vi "CalculateHaversineDirection.vi"(10 "Target Waypoint":cluster{"Longitude":dbl, "Latitude":dbl} {"Latitude" format="%#_8g"}, 11 "Robot Position":cluster{"Longitude":dbl, "Latitude":dbl}) -> (2 "polar angle":dbl)   [LabVIEW 2011]
panel:
  out "Robot Latitude":dbl
  out "Robot Longitude":dbl
  out "Target Latitude":dbl
  out "Target Longitude":dbl
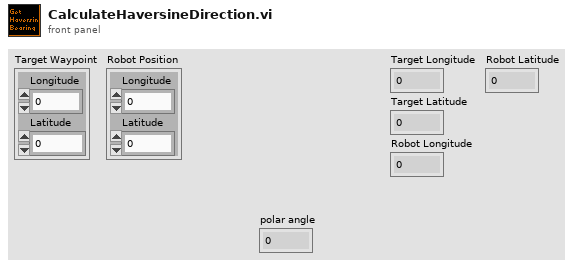
[diagram p1: front panel]
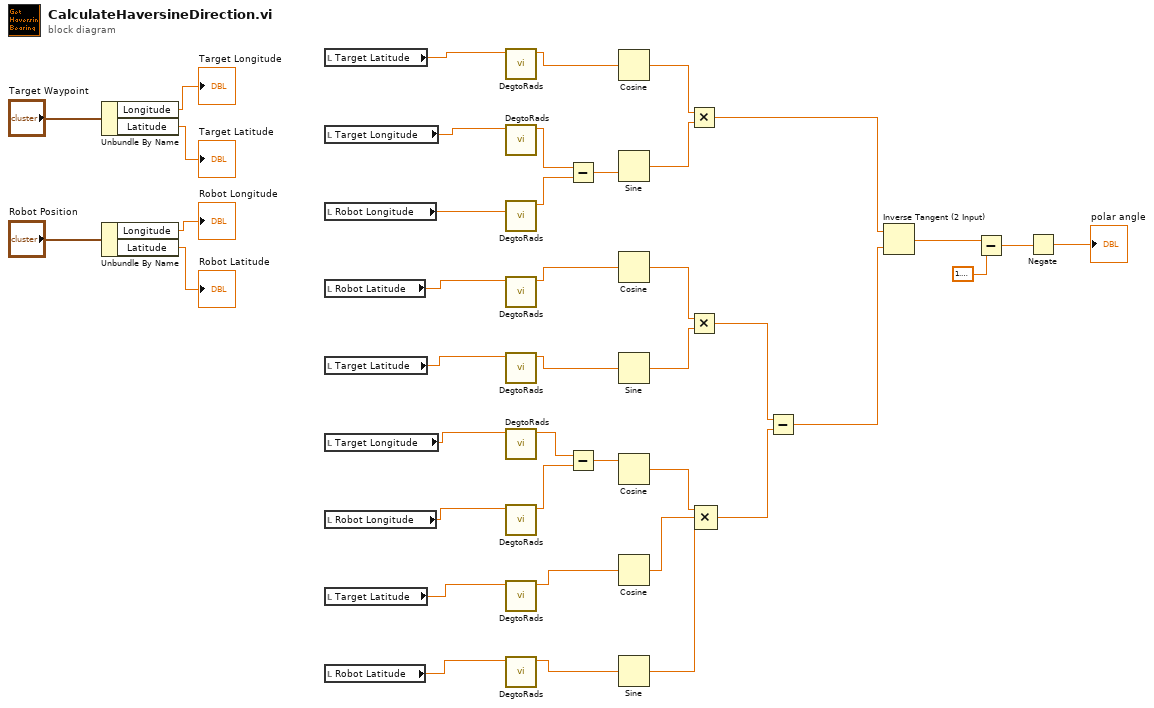
[diagram p0: block diagram]
diagram:
  n1 = Unbundle By Name("Target Waypoint") -> ("Longitude"=→"Target Longitude":dbl, "Latitude"=→"Target Latitude":dbl)
  n2 = Unbundle By Name("Robot Position") -> ("Longitude"=→"Robot Longitude":dbl, "Latitude"=→"Robot Latitude":dbl)
  n3 = local read "Target Latitude"() -> (w32:dbl)
  n4 = local read "Target Longitude"() -> (w31:dbl)
  n5 = local read "Robot Longitude"() -> (w30:dbl)
  n6 = local read "Robot Latitude"() -> (w33:dbl)
  n7 = local read "Target Latitude"() -> (w21:dbl)
  n8 = local read "Target Longitude"() -> (w35:dbl)
  n9 = local read "Robot Longitude"() -> (w34:dbl)
  n10 = local read "Target Latitude"() -> (w16:dbl)
  n11 = local read "Robot Latitude"() -> (w15:dbl)
  n12 = call "DegtoRads.vi"("Degrees in"=w32) -> ("Rads Out"=w24:dbl)  [unwired: 10 in]
  n13 = call "DegtoRads.vi"("Degrees in"=w31) -> ("Rads Out"=w29:dbl)  [unwired: 10 in]
  n14 = call "DegtoRads.vi"("Degrees in"=w30) -> ("Rads Out"=w28:dbl)  [unwired: 10 in]
  n15 = call "DegtoRads.vi"("Degrees in"=w33) -> ("Rads Out"=w20:dbl)  [unwired: 10 in]
  n16 = call "DegtoRads.vi"("Degrees in"=w21) -> ("Rads Out"=w19:dbl)  [unwired: 10 in]
  n17 = call "DegtoRads.vi"("Degrees in"=w35) -> ("Rads Out"=w27:dbl)  [unwired: 10 in]
  n18 = call "DegtoRads.vi"("Degrees in"=w34) -> ("Rads Out"=w26:dbl)  [unwired: 10 in]
  n19 = call "DegtoRads.vi"("Degrees in"=w16) -> ("Rads Out"=w14:dbl)  [unwired: 10 in]
  n20 = call "DegtoRads.vi"("Degrees in"=w15) -> ("Rads Out"=w13:dbl)  [unwired: 10 in]
  n21 = Subtract(x=w29, y=w28) -> (x-y=w25:dbl)
  n22 = Subtract(x=w27, y=w26) -> (x-y=w10:dbl)
  n23 = Cosine(x=w24) -> (cos(x)=w22:dbl)
  n24 = Sine(x=w25) -> (sin(x)=w23:dbl)
  n25 = Cosine(x=w20) -> (cos(x)=w17:dbl)
  n26 = Sine(x=w19) -> (sin(x)=w18:dbl)
  n27 = Cosine(x=w10) -> (cos(x)=w9:dbl)
  n28 = Cosine(x=w14) -> (cos(x)=w11:dbl)
  n29 = Sine(x=w13) -> (sin(x)=w12:dbl)
  n30 = Multiply(x=w22, y=w23) -> (x*y=w5:dbl)
  n31 = Multiply(x=w17, y=w18) -> (x*y=w7:dbl)
  n32 = Compound Arithmetic op=MULTIPLY(w9, w11, w12) -> (w8:dbl)
  n33 = Subtract(x=w7, y=w8) -> (x-y=w6:dbl)
  n34 = Inverse Tangent (2 Input)(1:w6, 2:w5) -> (0:w3:dbl)
  n35 = Subtract(x=w3, y=1.5707963267948966) -> (x-y=w2:dbl)
  n36 = Negate(x=w2) -> (-x=→"polar angle":dbl)
